vi "Find which point.vi"(5 "Direction":string(combo)="Forward", 7 "Choose":string(combo)="Less", 9 "Start Index":i32, 10 "y":dbl, 11 "Xn-Xn-1":dbl[](array[numeric])) -> (3 "Index":i32)   [LabVIEW 2021]
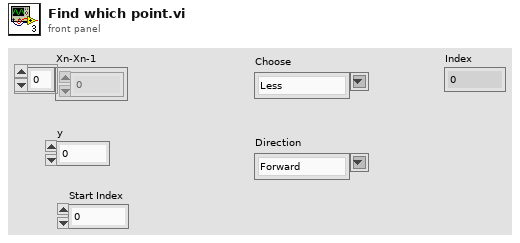
[diagram p1: front panel]
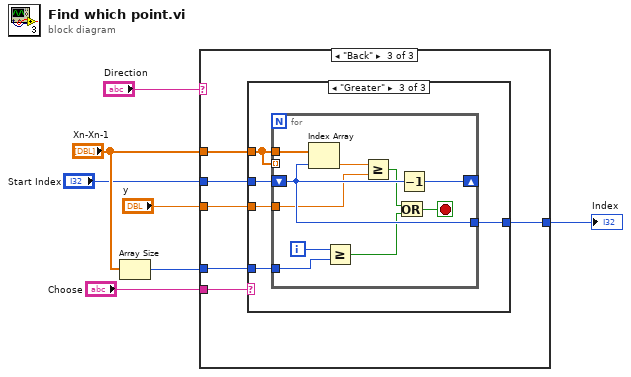
[diagram p0: block diagram]
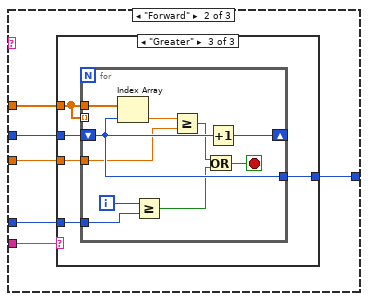
[diagram p3: hidden frame]
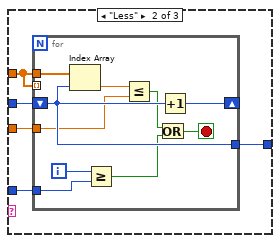
[diagram p5: hidden frame]
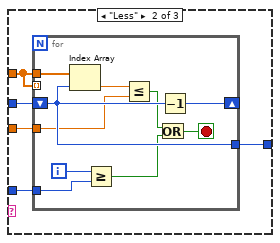
[diagram p7: hidden frame]
diagram:
  n1 = Array Size(array="Xn-Xn-1") -> (size(s)=w7:i32)
  n2 = case shown="\"Back\"" "Direction" {
    tunnel: w7 -> [_ w13 w49]
    tunnel: "Xn-Xn-1" -> [_ w12 w48]
    tunnel: "Start Index" -> [_ w11 w47]
    tunnel: "Choose" -> [_ w10 w46]
    tunnel: [_ w9 w45] -> w3
    tunnel: "y" -> [_ w8 w44]
    frame Default {
    }
    frame "Forward" {
      n3 = case shown="\"Greater\"" w10 {
        tunnel: w13 -> [_ w18 w33]
        tunnel: w12 -> [_ w17 w32]
        tunnel: w11 -> [_ w16 w31]
        tunnel: [_ w15 w30] -> w9
        tunnel: w8 -> [_ w14 w29]
        frame Default {
        }
        frame "Less" {
          n4 = for {
            tunnel: w17 -> [w28]
            shift-right: [w27] -> _
            shift-left: w16 -> [w26]
            tunnel: [w26] -> w15
            tunnel: w18 -> [w24]
            tunnel: w17 -> [_] mode=indexing
            tunnel: w14 -> [w19]
            i -> [w25]
            stop <- w21 stop-if-true
            n5 = Index Array(array=w28, index=w26) -> (element=w20:dbl)
            n6 = Greater Or Equal?(x=w25, y=w24) -> (x >= y?=w22:bool)
            n7 = Less Or Equal?(x=w20, y=w19) -> (x <= y?=w23:bool)
            n8 = Or(x=w23, y=w22) -> (x .or. y?=w21:bool)
            n9 = Increment(x=w26) -> (x+1=w27:i32)
          }
        }
        frame "Greater" {
          n10 = for {
            tunnel: w32 -> [w43]
            shift-right: [w42] -> _
            shift-left: w31 -> [w41]
            tunnel: [w41] -> w30
            tunnel: w33 -> [w39]
            tunnel: w32 -> [_] mode=indexing
            tunnel: w29 -> [w34]
            i -> [w40]
            stop <- w36 stop-if-true
            n11 = Index Array(array=w43, index=w41) -> (element=w35:dbl)
            n12 = Greater Or Equal?(x=w40, y=w39) -> (x >= y?=w37:bool)
            n13 = Greater Or Equal?(x=w35, y=w34) -> (x >= y?=w38:bool)
            n14 = Or(x=w38, y=w37) -> (x .or. y?=w36:bool)
            n15 = Increment(x=w41) -> (x+1=w42:i32)
          }
        }
      }
    }
    frame "Back" {
      n16 = case shown="\"Greater\"" w46 {
        tunnel: w49 -> [_ w54 w69]
        tunnel: w48 -> [_ w53 w68]
        tunnel: w47 -> [_ w52 w67]
        tunnel: [_ w51 w66] -> w45
        tunnel: w44 -> [_ w50 w65]
        frame Default {
        }
        frame "Less" {
          n17 = for {
            tunnel: w53 -> [w64]
            shift-right: [w63] -> _
            shift-left: w52 -> [w62]
            tunnel: [w62] -> w51
            tunnel: w54 -> [w60]
            tunnel: w53 -> [_] mode=indexing
            tunnel: w50 -> [w55]
            i -> [w61]
            stop <- w57 stop-if-true
            n18 = Index Array(array=w64, index=w62) -> (element=w56:dbl)
            n19 = Greater Or Equal?(x=w61, y=w60) -> (x >= y?=w58:bool)
            n20 = Less Or Equal?(x=w56, y=w55) -> (x <= y?=w59:bool)
            n21 = Or(x=w59, y=w58) -> (x .or. y?=w57:bool)
            n22 = Decrement(x=w62) -> (x-1=w63:i32)
          }
        }
        frame "Greater" {
          n23 = for {
            tunnel: w68 -> [w79]
            shift-right: [w78] -> _
            shift-left: w67 -> [w77]
            tunnel: [w77] -> w66
            tunnel: w69 -> [w75]
            tunnel: w68 -> [_] mode=indexing
            tunnel: w65 -> [w70]
            i -> [w76]
            stop <- w72 stop-if-true
            n24 = Index Array(array=w79, index=w77) -> (element=w71:dbl)
            n25 = Greater Or Equal?(x=w76, y=w75) -> (x >= y?=w73:bool)
            n26 = Greater Or Equal?(x=w71, y=w70) -> (x >= y?=w74:bool)
            n27 = Or(x=w74, y=w73) -> (x .or. y?=w72:bool)
            n28 = Decrement(x=w77) -> (x-1=w78:i32)
          }
        }
      }
    }
  }
  "Index" <- w3
